vi "demo - xy graph.vi"() -> ()   [LabVIEW 2024]
doc: "#vi_description \nPlot a constant phase sine wave against a sine wave with increase phase onto an XY graph.\nThetic Engineering Ltd."
uses:
  <vilib>/measure/NI_MABase.lvlib
  <vilib>/Analysis/NI_AALPro.lvlib
panel:
  in  "Stop":bool
  out "Phase":dbl(knob) scale=0.0..360.0
  in  "Amplitude":dbl(knob)=4.158804911152275 min=1.0 max=10.0 step=1.0 scale=1.0..10.0
  in  "Frequency":dbl(knob)=1.0 min=1.0 max=10.0 step=0.25 scale=1.0..10.0
  out "XY Graph":cluster{"Y":dbl[], "Y":dbl[]}(graph)
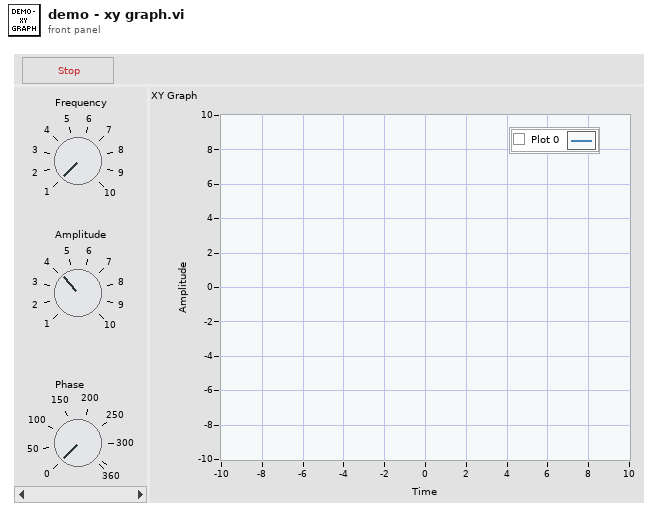
[diagram p1: front panel]
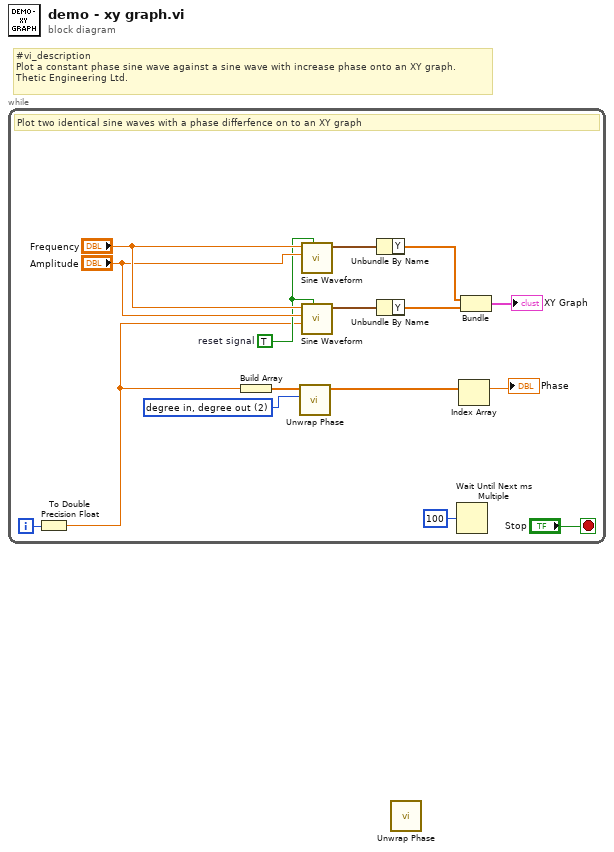
[diagram p0: block diagram]
diagram:
  # "#vi_description \nPlot a constant phase sine wave against a sine wave with increase phase onto an XY graph.\nThetic Engineering Ltd."
  n1 = while {
    i -> [w6]
    stop <- "Stop" stop-if-true
    w3 = 2 items=["radian in, radian out", "radian in, degree out", "degree in, degree out", "degree in, radian out"] ("phase unit")
    w7 = TRUE  # reset signal
    # "Plot two identical sine waves with a phase differfence on to an XY graph"
    n2 = To Double Precision Float(number=w6) -> (double precision float=w5:dbl)
    n3 = Build Array(w5) -> (w4:dbl[])
    n4 = call <vilib>:"Unwrap Phase.vi"("phase unit"=w3, "Phase"=w4) -> ("Unwrapped Phase"=w2:dbl[])  [unwired: 8 in, 1 out]
    n5 = call <vilib>:"Sine Waveform.vi"("reset signal"=w7, "amplitude"="Amplitude", "frequency"="Frequency") -> ("signal out"=w14:waveform(dbl))  [unwired: 7 in, 1 out]
    n6 = call <vilib>:"Sine Waveform.vi"("reset signal"=w7, "phase"=w5, "amplitude"="Amplitude", "frequency"="Frequency") -> ("signal out"=w13:waveform(dbl))  [unwired: 6 in, 1 out]
    n7 = Unbundle By Name(w14) -> ("Y"=w11:dbl[])
    n8 = Unbundle By Name(w13) -> ("Y"=w12:dbl[])
    n9 = Wait Until Next ms Multiple(millisecond multiple=u32 100) -> ()  [unwired: 1 out]
    n10 = Index Array(array=w2) -> (element=→"Phase":dbl)  [unwired: 1 in]
    n11 = Bundle("Y"=w11, "Y"=w12) -> (→"XY Graph":cluster{"Y":dbl[], "Y":dbl[]})  [unwired: 1 in]
  }
  n12 = call <vilib>:"Unwrap Phase.vi"() -> ()  [unwired: 10 in, 2 out]
